vi "模式三.vi"() -> ()   [LabVIEW 2014]
panel:
  in  "投彈按鈕":bool
  out "經過時間":dbl
  out "說明":string="本專題參考常見高中物理題型以及HW4。\n有一架轟炸機與一汽車水平距離為S0，轟炸機距離與地面維持高度H並保持固定速度Va水平飛行，汽車速度固定為Vc，請問轟炸機飛行多久後投彈可以命中汽車?Va、Vc、S0、H皆為變數，重力加速度為9.81，本程式會將時間點算出，並以動態圖示意。"
  out "車車":T1=TRUE
  out "合格":bool
  out "投彈時間(正解)":dbl
  in  "stop":bool
  in  "開始":bool
  out "Va":dbl=120.0
  out "Vc":dbl=30.0
  out "H":dbl=122.5
  out "S0":i32=630
  out "轟炸機":T2=TRUE
  out "String":string
  out "炸彈":T3=TRUE
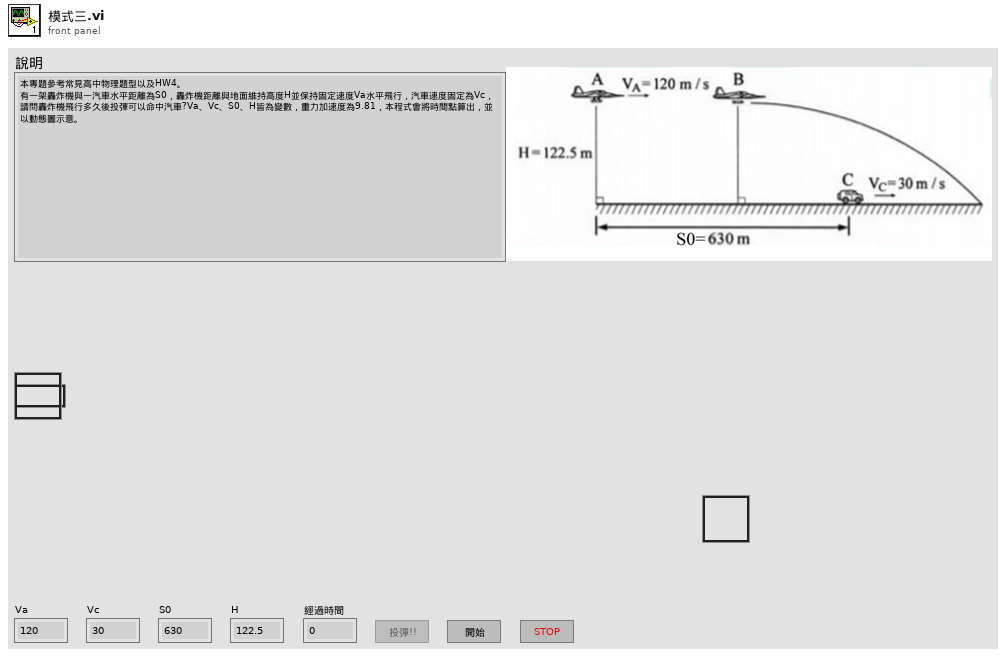
[diagram p1: front panel]
types:
  T1 = typedef "車!!.ctl" = bool
  T2 = typedef "飛機.ctl" = bool
  T3 = typedef "炸彈.ctl" = bool
  T4 = enum8{"Enabled", "Disabled", "Disabled and Grayed Out"}
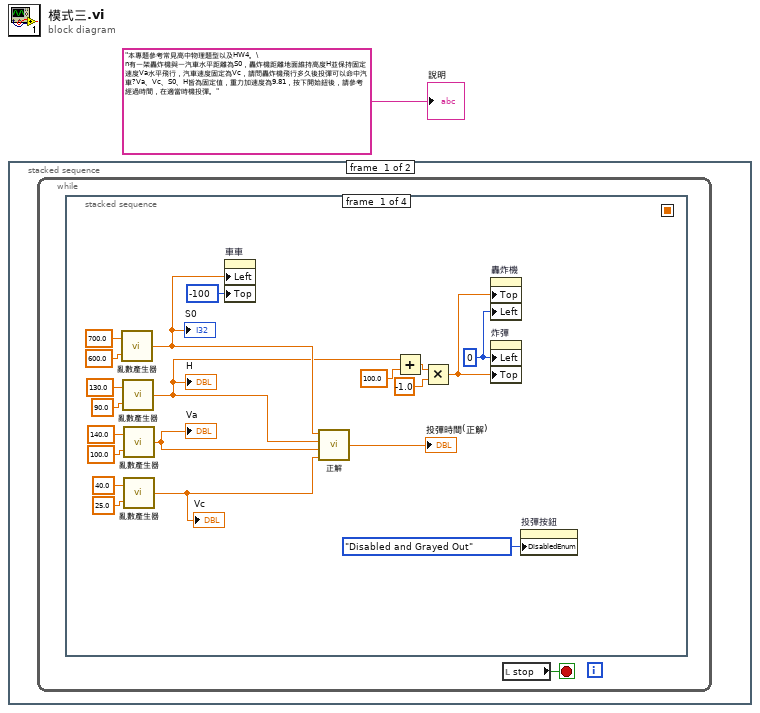
[diagram p0: block diagram]
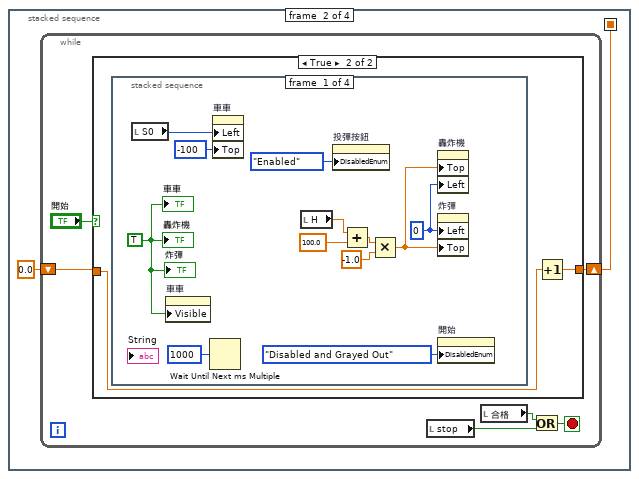
[diagram p2: hidden frame]
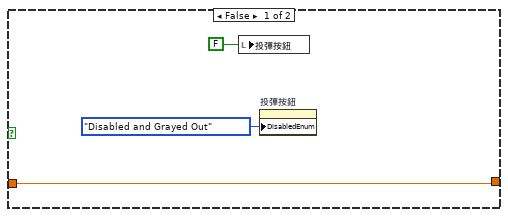
[diagram p3: hidden frame]
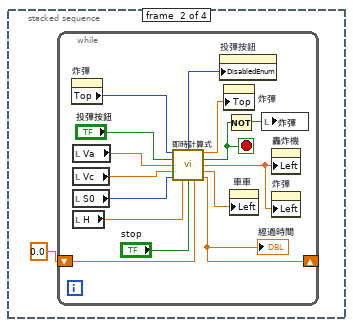
[diagram p4: hidden frame]
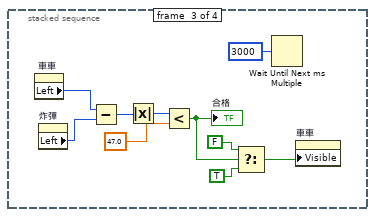
[diagram p5: hidden frame]
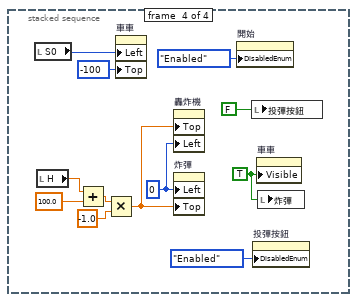
[diagram p6: hidden frame]
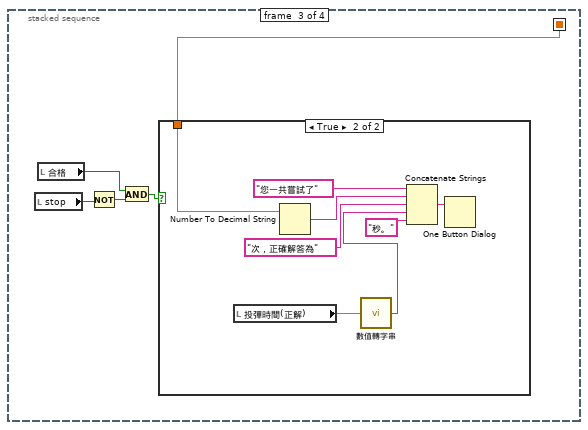
[diagram p7: hidden frame]
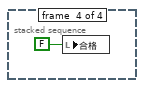
[diagram p9: hidden frame]
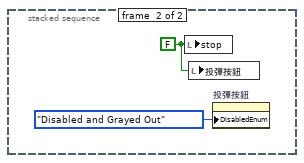
[diagram p10: hidden frame]
diagram:
  n1 = stacked-sequence {
    frame #0 {
      n2 = while {
        stop <- w2 stop-if-true
        n3 = stacked-sequence {
          seq-local: [_ w23 _ _] -> [_ _ w90 _]
          frame #0 {
            w7 = 0 ("Position:Left")
            n4 = call "亂數產生器.vi"("Min"=600.0, "Max"=700.0) -> ("Random"=w5:dbl)
            "S0" <- w5
            n5 = call "亂數產生器.vi"("Min"=90.0, "Max"=130.0) -> ("Random"=w4:dbl)
            "H" <- w4
            n6 = call "亂數產生器.vi"("Min"=100.0, "Max"=140.0) -> ("Random"=w13:dbl)
            "Va" <- w13
            n7 = call "亂數產生器.vi"("Min"=25.0, "Max"=40.0) -> ("Random"=w12:dbl)
            "Vc" <- w12
            n8 = property on="車車" class="Bool (strict)"("Left"=w5, "Top"=-100 ("Position:Top")) -> ()  [unwired: 2 in, 2 out]
            n9 = call "正解.vi"("Vc"=w12, "Va"=w13, "H"=w4, "S0"=w5) -> ("投彈時間(k)"=→"投彈時間(正解)":dbl)
            n10 = Add(x=w4, y=100.0) -> (x+y=w9:dbl)
            n11 = Multiply(x=w9, y=-1.0) -> (x*y=w8:dbl)
            n12 = property on="轟炸機" class="Bool (strict)"("Top"=w8, "Left"=w7) -> ()  [unwired: 2 in, 2 out]
            n13 = property on="炸彈" class="Bool (strict)"("Left"=w7, "Top"=w8) -> ()  [unwired: 2 in, 2 out]
            n14 = property on="投彈按鈕" class="Bool (strict)"("DisabledEnum"=T4."Disabled and Grayed Out" ("Disabled")) -> ()  [unwired: 2 in, 2 out]
          }
          frame #1 {
            n15 = while {
              shift-right: [w29] -> w23
              shift-left: 0.0 -> [w28]
              stop <- w25 stop-if-true
              n16 = case shown="True" "開始" {
                tunnel: w28 -> [w33 w35]
                tunnel: [w33 w34] -> w29
                frame False {
                  n17 = local write "投彈按鈕"(T3 FALSE ("炸彈")) -> ()
                  n18 = property on="投彈按鈕" class="Bool (strict)"("DisabledEnum"=T4."Disabled and Grayed Out" ("Disabled")) -> ()  [unwired: 2 in, 2 out]
                }
                frame True {
                  n19 = stacked-sequence {
                    frame #0 {
                      w40 = 0 ("Position:Left")
                      w37 = TRUE
                      n20 = local read "S0"() -> (w46:i32)
                      n21 = property on="車車" class="Bool (strict)"("Visible"=w37) -> ()  [unwired: 2 in, 2 out]
                      n22 = Wait Until Next ms Multiple(millisecond multiple=u32 1000) -> ()  [unwired: 1 out]
                      n23 = property on="車車" class="Bool (strict)"("Left"=w46, "Top"=-100 ("Position:Top")) -> ()  [unwired: 2 in, 2 out]
                      n24 = local read "H"() -> (w38:dbl)
                      n25 = property on="投彈按鈕" class="Bool (strict)"("DisabledEnum"=T4."Enabled" ("Disabled")) -> ()  [unwired: 2 in, 2 out]
                      n26 = Add(x=w38, y=100.0) -> (x+y=w42:dbl)
                      n27 = Multiply(x=w42, y=-1.0) -> (x*y=w41:dbl)
                      n28 = property on="轟炸機" class="Bool (strict)"("Top"=w41, "Left"=w40) -> ()  [unwired: 2 in, 2 out]
                      n29 = property on="炸彈" class="Bool (strict)"("Left"=w40, "Top"=w41) -> ()  [unwired: 2 in, 2 out]
                      n30 = property on="開始" class="Bool"("DisabledEnum"=T4."Disabled and Grayed Out" ("Disabled")) -> ()  [unwired: 2 in, 2 out]
                      "車車" <- w37
                      "轟炸機" <- w37
                      "炸彈" <- w37
                    }
                    frame #1 {
                      n31 = while {
                        shift-right: [w50] -> _
                        shift-left: 0.0 -> [w58]
                        stop <- w53 stop-if-true
                        n32 = property on="炸彈" class="Bool (strict)"() -> ("Top"=w63:i32)  [unwired: 2 in, 2 out]
                        n33 = local read "Va"() -> (w62:dbl)
                        n34 = local read "Vc"() -> (w61:dbl)
                        n35 = local read "S0"() -> (w60:i32)
                        n36 = local read "H"() -> (w59:dbl)
                        n37 = call "即時計算式.vi"("b y"=w63, "OK Button"="投彈按鈕", "Va"=w62, "Vc"=w61, "S0"=w60, "H"=w59, "stop"="stop", "ti"=w58) -> ("Disabled"=w49:T4, "b y 2"=w57:dbl, "output stop"=w53:bool, "a x"=w56:dbl, "c x"=w55:dbl, "to"=w50:dbl)  [unwired: 2 in]
                        "經過時間" <- w50
                        n38 = property on="投彈按鈕" class="Bool (strict)"("DisabledEnum"=w49) -> ()  [unwired: 2 in, 2 out]
                        n39 = property on="炸彈" class="Bool (strict)"("Top"=w57) -> ()  [unwired: 2 in, 2 out]
                        n40 = Not(x=w53) -> (.not. x?=w52:bool)
                        n41 = property on="車車" class="Bool (strict)"("Left"=w55) -> ()  [unwired: 2 in, 2 out]
                        n42 = local write "炸彈"(w52) -> ()
                        n43 = property on="轟炸機" class="Bool (strict)"("Left"=w56) -> ()  [unwired: 2 in, 2 out]
                        n44 = property on="炸彈" class="Bool (strict)"("Left"=w56) -> ()  [unwired: 2 in, 2 out]
                      }
                    }
                    frame #2 {
                      n45 = property on="車車" class="Bool (strict)"() -> ("Left"=w69:i32)  [unwired: 2 in, 2 out]
                      n46 = property on="炸彈" class="Bool (strict)"() -> ("Left"=w73:i32)  [unwired: 2 in, 2 out]
                      n47 = Subtract(x=w69, y=w73) -> (x-y=w72:i32)
                      n48 = Absolute Value(x=w72) -> (abs(x)=w71:i32)
                      n49 = Less?(x=w71, y=47.0) -> (x < y?=w68:bool)
                      "合格" <- w68
                      n50 = Select(t=FALSE, s=w68, f=TRUE) -> (s? t:f=w67:bool)
                      n51 = Wait Until Next ms Multiple(millisecond multiple=u32 3000) -> ()  [unwired: 1 out]
                      n52 = property on="車車" class="Bool (strict)"("Visible"=w67) -> ()  [unwired: 2 in, 2 out]
                    }
                    frame #3 {
                      w76 = TRUE ("Visible")
                      w79 = 0 ("Position:Left")
                      n53 = local read "S0"() -> (w83:i32)
                      n54 = local read "H"() -> (w77:dbl)
                      n55 = Add(x=w77, y=100.0) -> (x+y=w81:dbl)
                      n56 = Multiply(x=w81, y=-1.0) -> (x*y=w80:dbl)
                      n57 = property on="車車" class="Bool (strict)"("Left"=w83, "Top"=-100 ("Position:Top")) -> ()  [unwired: 2 in, 2 out]
                      n58 = property on="轟炸機" class="Bool (strict)"("Top"=w80, "Left"=w79) -> ()  [unwired: 2 in, 2 out]
                      n59 = property on="炸彈" class="Bool (strict)"("Left"=w79, "Top"=w80) -> ()  [unwired: 2 in, 2 out]
                      n60 = property on="開始" class="Bool"("DisabledEnum"=T4."Enabled" ("Disabled")) -> ()  [unwired: 2 in, 2 out]
                      n61 = local write "投彈按鈕"(T3 FALSE ("炸彈")) -> ()
                      n62 = property on="投彈按鈕" class="Bool (strict)"("DisabledEnum"=T4."Enabled" ("Disabled")) -> ()  [unwired: 2 in, 2 out]
                      n63 = property on="車車" class="Bool (strict)"("Visible"=w76) -> ()  [unwired: 2 in, 2 out]
                      n64 = local write "炸彈"(w76) -> ()
                    }
                  }
                  n65 = Increment(x=w35) -> (x+1=w34:dbl)
                }
              }
              n66 = local read "stop"() -> (w26:bool)
              n67 = local read "合格"() -> (w27:bool)
              n68 = Or(x=w27, y=w26) -> (x .or. y?=w25:bool)
            }
          }
          frame #2 {
            n69 = local read "stop"() -> (w89:bool)
            n70 = local read "合格"() -> (w86:bool)
            n71 = Not(x=w89) -> (.not. x?=w87:bool)
            n72 = And(x=w86, y=w87) -> (x .and. y?=w88:bool)
            n73 = case shown="True" w88 {
              tunnel: w90 -> [_ w91]
              frame False {
              }
              frame True {
                n74 = local read "投彈時間(正解)"() -> (w94:dbl)
                n75 = Number To Decimal String(number=w91) -> (decimal integer string=w96:string)  [unwired: 1 in]
                n76 = call "數值轉字串.vi"("number"=w94) -> ("s? t:f"=w93:string)
                n77 = Concatenate Strings("您一共嘗試了" ("string"), w96, "次，正確解答為" ("string"), w93, "秒。" ("string")) -> (w98:string)
                n78 = One Button Dialog(message=w98) -> ()  [unwired: 1 in, 1 out]
              }
            }
          }
          frame #3 {
            n79 = local write "合格"(FALSE) -> ()
          }
        }
        n80 = local read "stop"() -> (w2:bool)
      }
    }
    frame #1 {
      w100 = FALSE ("stop")
      n81 = local write "stop"(w100) -> ()
      n82 = local write "投彈按鈕"(w100) -> ()
      n83 = property on="投彈按鈕" class="Bool (strict)"("DisabledEnum"=T4."Disabled and Grayed Out" ("Disabled")) -> ()  [unwired: 2 in, 2 out]
    }
  }
  "說明" <- "本專題參考常見高中物理題型以及HW4。\n有一架轟炸機與一汽車水平距離為S0，轟炸機距離地面維持高度H並保持固定速度Va水平飛行，汽車速度固定為Vc，請問轟炸機飛行多久後投彈可以命中汽車?Va、Vc、S0、H皆為固定值，重力加速度為9.81，按下開始鈕後，請參考經過時間，在適當時機投彈。" ("說明")
